vi "Motion_xbee_1Radar.vi"(0 "VISA resource name":refnum<visa-resource-name>="COM1", 1 "baud rate":u32=9600, 4 "data bits":u16=8 min=5 max=8 step=1, 5 "parity":u16(ring) items=["None", "Odd", "Even", "Mark", "Space"], 7 "stop bits":u16=10, 9 "XON Character":u8=17 format="%.0x", 14 "XOFF Character":u8=19 format="%.0x", 15 "timeout (ms)":u32=10000, 21 "End read on termination character?":bool, 24 "termination char\n(0xA = '\\n' = LF)":u8=10 format="%.0x", 25 "buffer size":u32=4096) -> ()   [LabVIEW 2015]
doc: "The Advanced Serial Read and Write example performs a Serial Port Read, a Serial Port Write, or a combination of these actions while setting some advanced serial features like buffer size, termination characters, and XON/XOFF flow control. The user selects the actions (read or write) on the front panel. If both are selected, the VI will write the data first, read the data and then close the VISA session that is opened to the port. \n\nThe parameters set for the serial port must match the parameters of the connected instrument or device. In this example, the bytes to read parameter specifies the number of bytes that the serial port reads. If there were more bytes at the port than the number specified in bytes to read, those bytes would not be read. Also, if you specify to read more bytes than the number of bytes actually read, you might receive a timeout error message.\n\nINSTRUCTIONS:\n1) Select the serial resource and configuration parameters (baud rate, data bits, parity, stop bits, flow control).\n2) Termination character can be enabled and set. Also, set the required input buffer size prior to running the example.\n3) Select the operations to be performed. \n4) Connect the serial port to your device. If no device is available, perform a loopback test by doing one of the following. Short pins 2 and 3 on a RS-232 cable or short pin 4 to pin 8 and pin 5 to pin 9 on a RS-485/422 cable. \n5) Run the VI to see the data read. (The \"read string\" will match the \"string to write\" if a loopback test was performed.)\n\nThis example exposes several advanced features that you may need for your application. Not all applications need all the features shown in this example. The input buffer size is likely an important setting that you want to control in your application. This example expands upon the flow control option for XON and XOFF, allowing the user to choose those control characters. The timeout parameter has been brought to the front panel so a user can specify the time period the VISA Read will wait for the number of bytes to read before timing out. Also, the user has several controls for the termination character, which is discussed later.\n\nNote that you can press the write and read buttons and change the bytes to read parameters on the fly, while the example is running. However, you must stop the example to change the other configuration parameters after the example has started running, and then run again.\n\nSet the I/O buffer size slightly higher the amount of data you expect to receive. This is very important for applications that don't use flow control, as you may lose characters if the receive buffer overflows.\n\nSetting the timeout period ensures that the operation returns with a timeout error if the operation cannot be performed in the specified time period. \n\nSome devices require a termination character in order to identify the end of command strings. Some devices send a termination character to signify the end of data to be read. \n\nThis example shows how you can end the Read operation once a termination character is detected in the buffer and/or append a termination character at the end of the Write data. To enable the Read to end on a termination character, use the VISA Configure Serial Port or use the VISA Properties Serial End Mode for Reads, Termination Character Enable, and Termination Character. To end the Write with a termination character, use the VISA Properties Serial End Mode for Writes, the Send End Enable, and Termination Character. In this example, the same termination character is used for both the Read and the Write. You can specify two different characters for your application, if desired.\n\nYour application may require specific characters for the XON/XOFF Flow Control. You can specify these characters with the VISA Properties Flow Control XOFF Character and Flow Control XON Character. Note that if the standard XON and XOFF characters are used, then decimal 17 and 19 are unavailable for data values. Remember that using flow control and setting an adequate buffer size allow you to prevent buffer overflows."
uses:
  <vilib>/Analysis/2dsp.llb/Complex FFT.vi
  <vilib>/Instr/_visa.llb/VISA Configure Serial Port (Instr).vi
  <vilib>/measure/madcrms.llb/Basic Averaged DC-RMS for 1 Chan.vi
  <vilib>/measure/NI_MAPro.lvlib
  <vilib>/Analysis/NI_AALPro.lvlib
panel:
  in  "Data saving path":path=path "C:/Users/zpeng/OneDrive - Texas Tech University/Desktop"
  in  "Save raw data":bool
  out "Spectrum":waveform(dbl)(graph)
  out "I/Q channels":dynamicdata(graph)
  in  "time":timestamp=timestamp(3198752888.296 s since 1904-01-01)
  in  "FFT":i32=256
  in  "flow control":u16(ring) items=["None"=0, "XON/XOFF"=1, "RTS/CTS"=2, "DTR/DSR"=4]
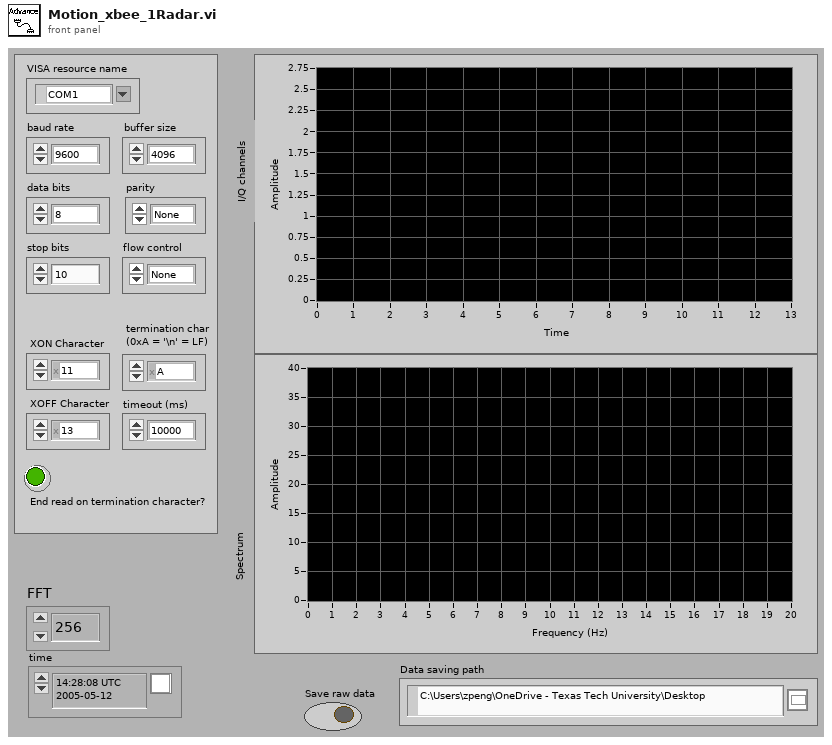
[diagram p1: front panel]
types:
  T1 = enum16{"open", "replace", "create", "open or create", "replace or create", "replace or create with confirmation"}
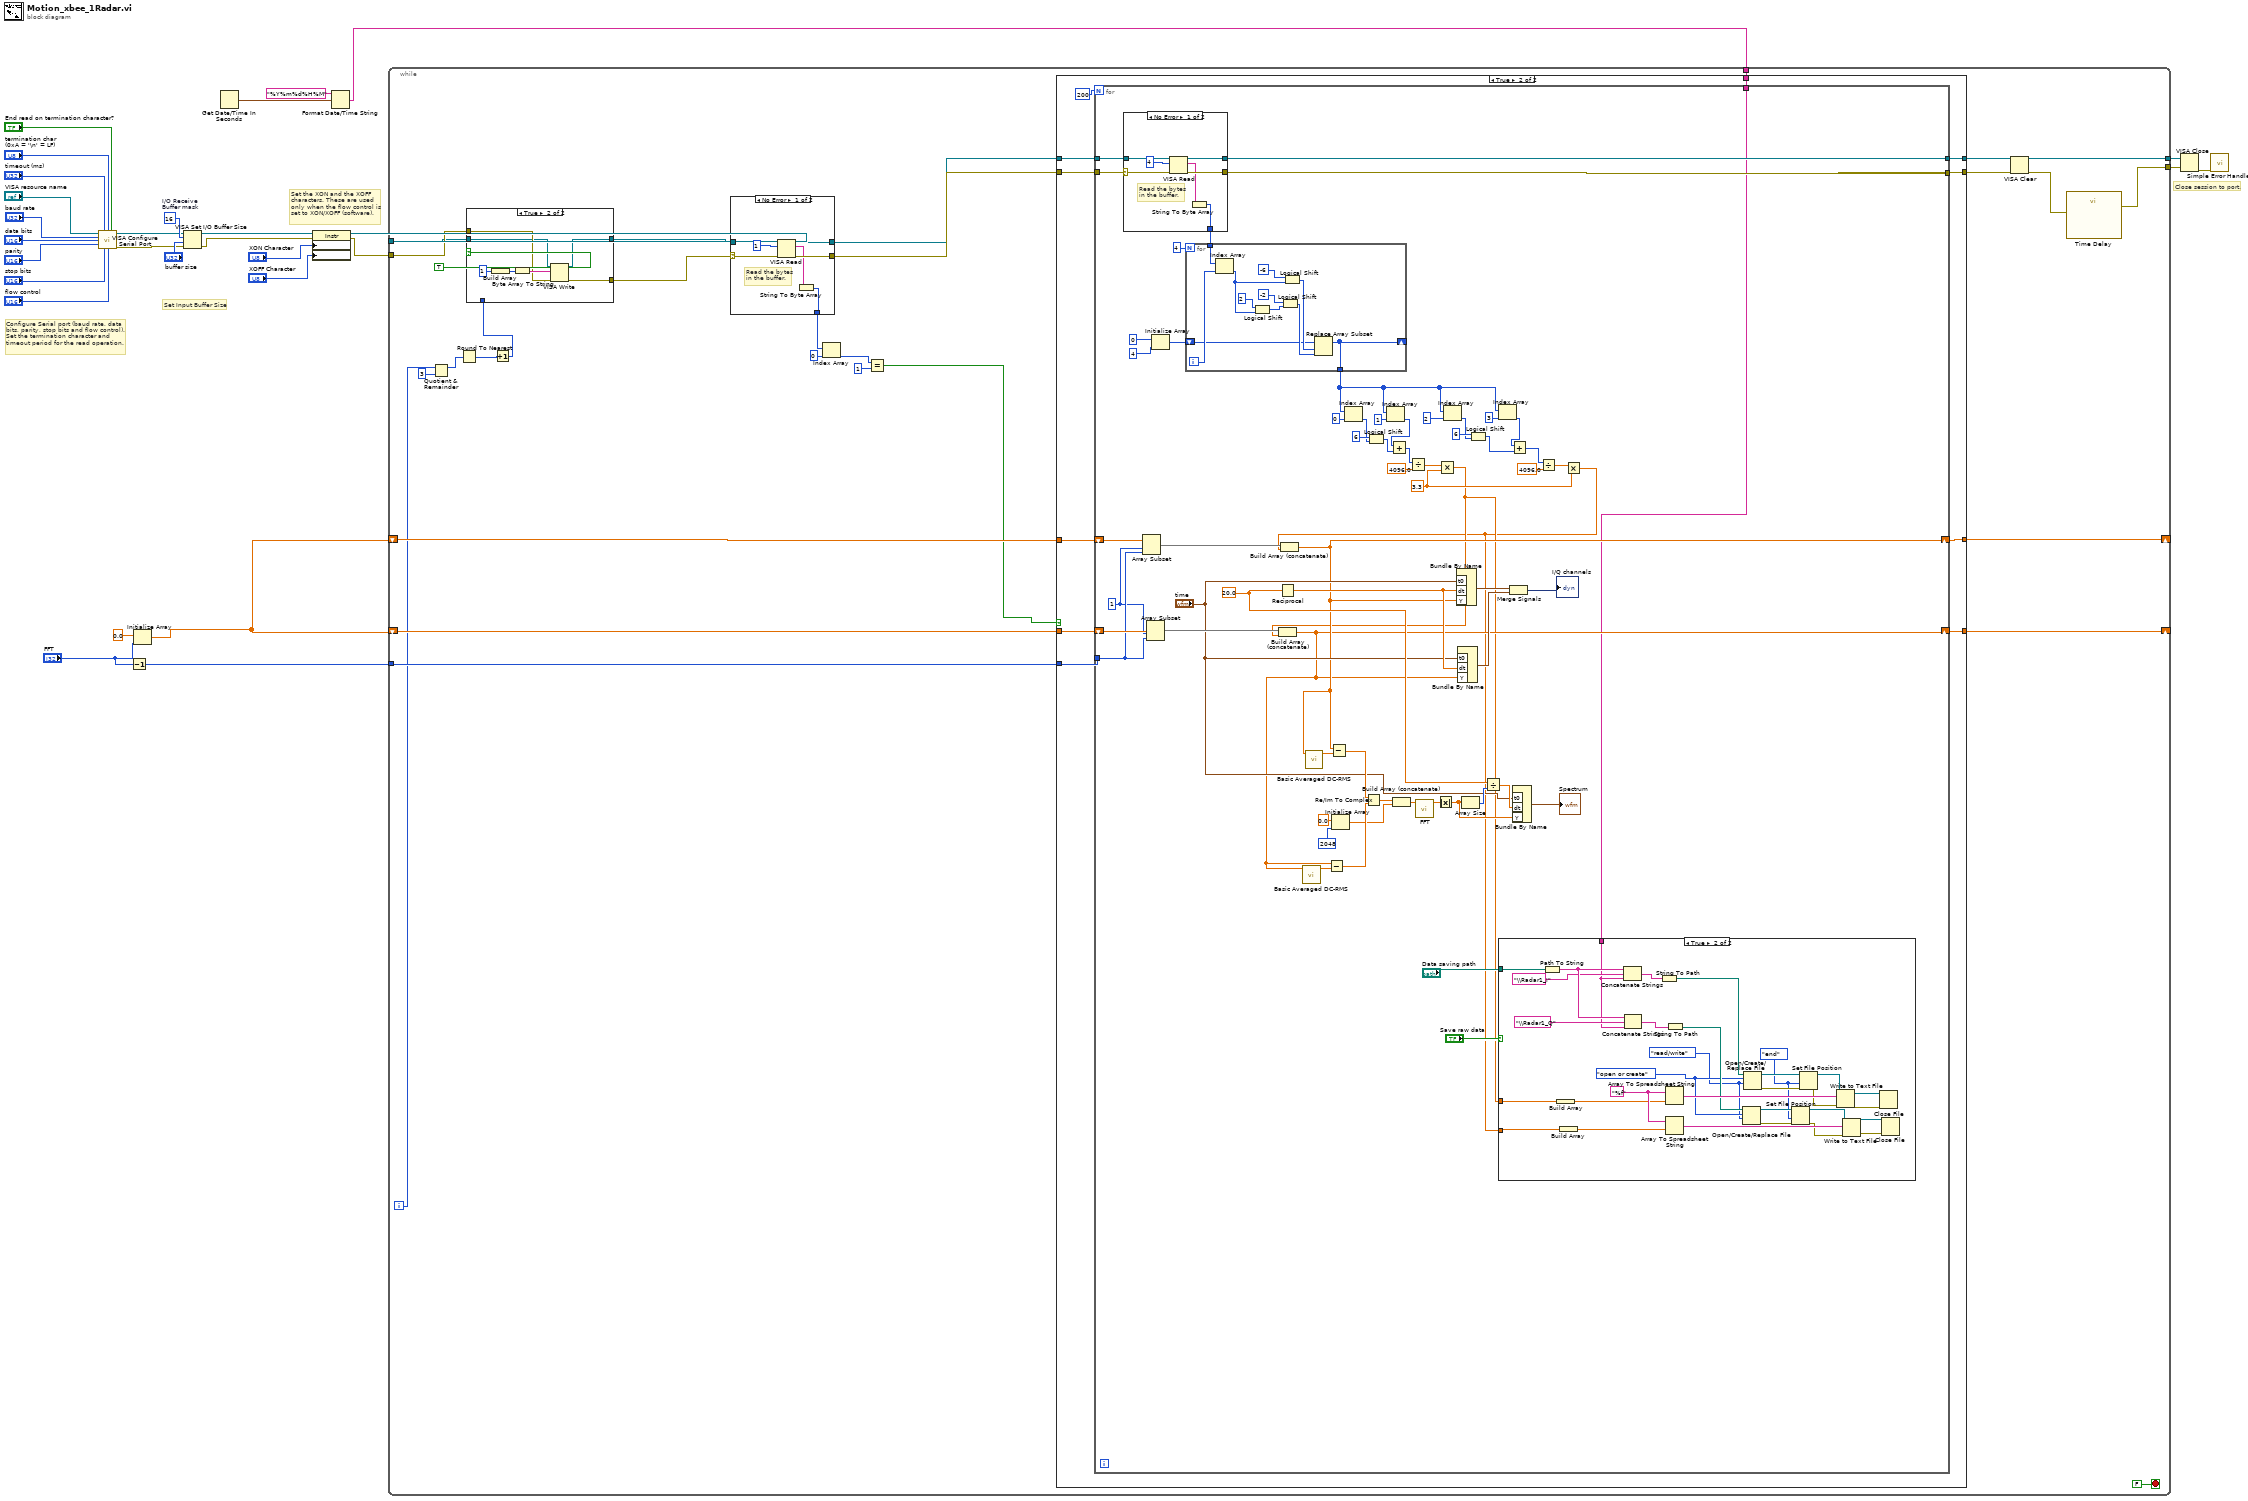
[diagram p0: block diagram]
diagram:
  w22 = u16 16  # I/O Receive Buffer mask
  # "Set the XON and the XOFF\ncharacters. These are used\nonly when the flow control is\nset to XON/XOFF (software)."
  # "Configure Serial port (baud rate, data\nbits, parity, stop bits and flow control).\nSet the termination character and\ntimeout period for the read operation."
  # "Set Input Buffer Size"
  # "Close session to port."
  n1 = call-poly "VISA Configure Serial Port"("VISA resource name"="VISA resource name", "timeout (10sec)"="timeout (ms)", "termination char\n(0xA = '\\n' = LF)"="termination char\n(0xA = '\\n' = LF)", "Enable Termination\nChar (T)"="End read on termination character?", "baud rate (9600)"="baud rate", "data bits (8)"="data bits", "parity (0:none)"="parity", "stop bits (10: 1 bit)"="stop bits", "flow control (0:none)"="flow control") -> ("VISA resource name out"=w8:refnum<visa-resource-name>, "error out"=w7:errorcluster)  [unwired: 1 in, 4 out]
  n2 = Decrement(x="FFT") -> (x-1=w11:i32)
  n3 = Initialize Array(0.0 ("element"), "FFT") -> (w6:dbl[])
  n4 = VISA Set I/O Buffer Size(VISA resource name=w8, mask (16)=w22, size (4096)="buffer size", error in (no error)=w7) -> (VISA resource name out=w18:refnum<visa-resource-name>, error out=w17:errorcluster)
  n5 = Get Date/Time In Seconds() -> (seconds since 1Jan1904=w2:timestamp)
  n6 = property class="Instr"(reference=w18, error in=w17, "Serial Settings:Flow Control XON Character"="XON Character", "Serial Settings:Flow Control XOFF Character"="XOFF Character") -> (reference out=w5:refnum<visa-resource-name>, error out=w4:errorcluster)
  n7 = Format Date/Time String(time format string (%c)="%Y%m%d%H%M", seconds (now)=w2) -> (date/time string=w1:string)  [unwired: 1 in]
  n8 = while {
    tunnel: w11 -> [w58]
    tunnel: w5 -> [w51]
    tunnel: [w45] -> w13
    tunnel: w4 -> [w52]
    tunnel: [w49] -> w12
    shift-right: [w53] -> _
    shift-left: w6 -> [w57]
    shift-right: [w54] -> _
    shift-left: w6 -> [w55]
    tunnel: w1 -> [w30]
    i -> [w34]
    stop <- FALSE stop-if-true
    n9 = Quotient & Remainder(x=w34, y=3) -> (x-y*floor(x/y)=w35:i32)  [unwired: 1 out]
    n10 = Round To Nearest(number=w35) -> (nearest integer value=w32:i32)
    n11 = Increment(x=w32) -> (x+1=w31:i32)
    n12 = case shown="True" TRUE {
      tunnel: w52 -> [w199 w205]
      tunnel: w51 -> [w198 w204]
      tunnel: [w198 w203] -> w43
      tunnel: [w199 w202] -> w44
      tunnel: w31 -> [_ _]
      frame False {
      }
      frame True {
        n13 = Build Array(u8 1 ("element")) -> (w201:u8[])
        n14 = Byte Array To String(unsigned byte array=w201) -> (string=w206:string)
        n15 = VISA Write(VISA resource name=w204, write buffer=w206, error in (no error)=w205) -> (VISA resource name out=w203:refnum<visa-resource-name>, error out=w202:errorcluster)  [unwired: 1 out]
      }
    }
    n16 = case "Read bytes from port." shown="No Error" w44 {
      selector: w44 -> [w62 w67]
      tunnel: [w64 w67] -> w42
      tunnel: [w65 w68] -> w41
      tunnel: w43 -> [w63 w68]
      tunnel: [w60 u8[] [] ("unsigned byte array")] -> w40
      frame No Error {
        # "Read the bytes\nin the buffer."
        n17 = VISA Read(VISA resource name=w63, byte count=u32 1, error in (no error)=w62) -> (VISA resource name out=w65:refnum<visa-resource-name>, read buffer=w61:string, error out=w64:errorcluster)  [unwired: 1 out]
        n18 = String To Byte Array(string=w61) -> (unsigned byte array=w60:u8[])
      }
      frame Error {
        # "Error occurred \nreading Bytes at \nSerial Port"
      }
    }
    n19 = Index Array(array=w40, index=0) -> (element=w38:u8)
    n20 = Equal?(x=w38, y=u8 1) -> (x = y?=w36:bool)
    n21 = case shown="True" w36 {
      tunnel: w58 -> [_ w83]
      tunnel: w57 -> [w70 w81]
      tunnel: w55 -> [w69 w80]
      tunnel: [w69 w79] -> w54
      tunnel: [w70 w78] -> w53
      tunnel: [w72 w77] -> w48
      tunnel: w41 -> [w72 w76]
      tunnel: w42 -> [w71 w75]
      tunnel: [w71 w74] -> w47
      tunnel: w30 -> [_ w73]
      frame False {
      }
      frame True {
        n22 = for {
          N: 200 -> [_]
          tunnel: w75 -> [w117]
          tunnel: w76 -> [w116]
          tunnel: [w91] -> w77
          tunnel: [w90] -> w74
          tunnel: w83 -> [w129]
          shift-right: [w96] -> w78
          shift-left: w81 -> [w144]
          shift-right: [w97] -> w79
          shift-left: w80 -> [w130]
          tunnel: w73 -> [w86]
          w98 = 1 ("index")
          (unwired) 0
          w122 = 3.3 ("y")
          w106 = 20.0 ("dt")
          n23 = case "Read bytes from port." shown="No Error" w117 {
            selector: w117 -> [w191 w196]
            tunnel: [w193 w196] -> w90
            tunnel: [w194 w197] -> w91
            tunnel: w116 -> [w192 w197]
            tunnel: [w189 u8[] [] ("unsigned byte array")] -> w92
            frame No Error {
              # "Read the bytes\nin the buffer."
              n24 = VISA Read(VISA resource name=w192, byte count=u32 4, error in (no error)=w191) -> (VISA resource name out=w194:refnum<visa-resource-name>, read buffer=w190:string, error out=w193:errorcluster)  [unwired: 1 out]
              n25 = String To Byte Array(string=w190) -> (unsigned byte array=w189:u8[])
            }
            frame Error {
              # "Error occurred \nreading Bytes at \nSerial Port"
            }
          }
          n26 = Array Subset(array=w130, index=w98, length=w129) -> (w131:dbl[])
          n27 = Array Subset(array=w144, index=w98, length=w129) -> (w145:dbl[])
          n28 = Initialize Array(i16 0 ("element"), 4 ("dimension size")) -> (w93:i16[])
          n29 = for {
            N: 4 -> [_]
            tunnel: w92 -> [w182]
            tunnel: [w177] -> w99
            shift-right: [w177] -> _
            shift-left: w93 -> [w178]
            i -> [w181]
            n30 = Index Array(array=w182, index=w181) -> (element=w185:u8)
            n31 = Logical Shift(y=i8 2, x=w185) -> (x << y=w184:u8)
            n32 = Logical Shift(y=i8 -2, x=w184) -> (x << y=w179:u8)
            n33 = Logical Shift(y=i8 -6, x=w185) -> (x << y=w180:u8)
            n34 = Replace Array Subset(array=w178, new element=w179, index=w180) -> (w177:i16[])
          }
          n35 = Reciprocal(x=w106) -> (1/x=w120:dbl)
          n36 = Initialize Array(0.0 ("element"), 2048 ("dimension size")) -> (w110:dbl[])
          n37 = Index Array(array=w99, index=0) -> (element=w138:i16)
          n38 = Logical Shift(y=i16 6, x=w138) -> (x << y=w134:i16)
          n39 = Index Array(array=w99, index=1) -> (element=w135:i16)
          n40 = Add(x=w135, y=w134) -> (x+y=w89:i16)
          n41 = Divide(x=w89, y=4096.0) -> (x/y=w127:dbl)
          n42 = Multiply(x=w127, y=w122) -> (x*y=w85:dbl)
          n43 = Build Array (concatenate)(w145, w85) -> (w96:dbl[])
          n44 = call-poly <vilib>:"Basic Averaged DC-RMS.vi"("signal in"=w96) -> ("DC value"=w123:dbl)  [unwired: 4 in, 6 out]
          n45 = Subtract(x=w96, y=w123) -> (x-y=w114:dbl[])
          n46 = Index Array(array=w99, index=2) -> (element=w136:i16)
          n47 = Bundle By Name ("Build Waveform")("t0"="time", "dt"=w120, "Y"=w96) -> (w118:waveform(dbl))  [unwired: 1 out]
          n48 = Logical Shift(y=i16 6, x=w136) -> (x << y=w132:i16)
          n49 = Index Array(array=w99, index=3) -> (element=w133:i16)
          n50 = Add(x=w133, y=w132) -> (x+y=w101:i16)
          n51 = Divide(x=w101, y=4096.0) -> (x/y=w125:dbl)
          n52 = Multiply(x=w125, y=w122) -> (x*y=w84:dbl)
          n53 = Build Array (concatenate)(w131, w84) -> (w97:dbl[])
          n54 = call-poly <vilib>:"Basic Averaged DC-RMS.vi"("signal in"=w97) -> ("DC value"=w124:dbl)  [unwired: 4 in, 6 out]
          n55 = Subtract(x=w97, y=w124) -> (x-y=w115:dbl[])
          n56 = Re/Im To Complex(1:w114, 2:w115) -> (0:w109:cdb[])
          n57 = Build Array (concatenate)(w109, w110) -> (w111:cdb[])
          n58 = call-poly <vilib>:"FFT.vi"("X"=w111) -> ("FFT {X}"=w107:cdb[])  [unwired: 2 in, 8 out]
          n59 = Absolute Value(x=w107) -> (abs(x)=w105:dbl[])
          n60 = Bundle By Name ("Build Waveform")("t0"="time", "dt"=w120, "Y"=w97) -> (w119:waveform(dbl))  [unwired: 1 out]
          n61 = Array Size(array=w105) -> (size(s)=w108:i32)
          n62 = Divide(x=w106, y=w108) -> (x/y=w104:dbl)
          n63 = case shown="True" "Save raw data" {
            tunnel: w85 -> [_ w166]
            tunnel: w84 -> [_ w147]
            tunnel: w86 -> [_ w168]
            tunnel: "Data saving path" -> [_ w167]
            frame False {
            }
            frame True {
              w148 = enum16{"read/write", "read-only", "write-only"}."read/write" ("access (0:read/write)")
              w149 = T1."open or create" ("operation (0:open)")
              w157 = enum16{"start", "end", "current"}."end" ("from (0:start)")
              w172 = "%f" ("format string")
              n64 = Path To String(path=w167) -> (string=w174:string)
              n65 = Build Array(w166) -> (w146:dbl[])
              n66 = Build Array(w147) -> (w165:dbl[])
              n67 = Concatenate Strings(w174, "\\Radar1_I" ("string"), w168) -> (w176:string)
              n68 = Concatenate Strings(w174, "\\Radar1_Q" ("string"), w168) -> (w173:string)
              n69 = String To Path(string=w176) -> (path=w164:path)
              n70 = Array To Spreadsheet String(array=w146, 3:w172) -> (spreadsheet string=w175:string)  [unwired: 1 in]
              n71 = Array To Spreadsheet String(array=w165, 3:w172) -> (spreadsheet string=w171:string)  [unwired: 1 in]
              n72 = String To Path(string=w173) -> (path=w163:path)
              n73 = Open/Create/Replace File(file path (use dialog)=w163, operation (0:open)=w149, access (0:read/write)=w148) -> (refnum out=w158:refnum<file>, error out=w156:errorcluster)  [unwired: 3 in, 1 out]
              n74 = Open/Create/Replace File(file path (use dialog)=w164, operation (0:open)=w149, access (0:read/write)=w148) -> (refnum out=w162:refnum<file>, error out=w161:errorcluster)  [unwired: 3 in, 1 out]
              n75 = Set File Position(refnum=w158, from (0:start)=w157, error in=w156) -> (refnum out=w154:refnum<file>, error out=w155:errorcluster)  [unwired: 1 in]
              n76 = Set File Position(refnum=w162, from (0:start)=w157, error in=w161) -> (refnum out=w160:refnum<file>, error out=w159:errorcluster)  [unwired: 1 in]
              n77 = Write to Text File(file (use dialog)=w160, text=w175, error in=w159) -> (refnum out=w153:refnum<file>, error out=w152:errorcluster)  [unwired: 1 in, 1 out]
              n78 = Write to Text File(file (use dialog)=w154, text=w171, error in=w155) -> (refnum out=w151:refnum<file>, error out=w150:errorcluster)  [unwired: 1 in, 1 out]
              n79 = Close File(refnum=w153, error in=w152) -> ()  [unwired: 2 out]
              n80 = Close File(refnum=w151, error in=w150) -> ()  [unwired: 2 out]
            }
          }
          n81 = Merge Signals(w119, w118) -> (→"I/Q channels":dynamicdata)
          n82 = Bundle By Name("t0"="time", "dt"=w104, "Y"=w105) -> (→"Spectrum":waveform(dbl))  [unwired: 1 out]
        }
      }
    }
    n83 = VISA Clear(VISA resource name=w48, error in (no error)=w47) -> (VISA resource name out=w45:refnum<visa-resource-name>, error out=w46:errorcluster)
    n84 = call "Time Delay"("error in (no error)"=w46) -> ("error out"=w49:errorcluster)  [unwired: 10 in]
  }
  n85 = VISA Close(VISA resource name=w13, error in (no error)=w12) -> (error out=w27:errorcluster)
  n86 = call <vilib>:"Simple Error Handler.vi"("error in (no error)"=w27) -> ()  [unwired: 1 in, 8 out]
